vi "LSM9DS1 IMU Example.vi"() -> ()   [LabVIEW 2020]
doc: "Example for reading from the LSM9DS1 9-axis IMU using the LINX toolkit."
uses:
  <vilib>/MakerHub/LINX/Public/Utilities/Open Local.vi
  LINX I2C/LINX I2C.lvclass
  <vilib>/MakerHub/LINX/LMH-LINX.lvlib
  LSM9DS1/LSM9DS1 IMU.lvclass
panel:
  out "Magnetometer":cluster{"x":dbl, "y":dbl, "z":dbl}(graph)
  out "Accelerometer":cluster{"x":dbl, "y":dbl, "z":dbl}(graph)
  in  "stop":bool
  out "Gyro":cluster{"x":dbl, "y":dbl, "z":dbl}(graph)
  out "Error Out":errorcluster
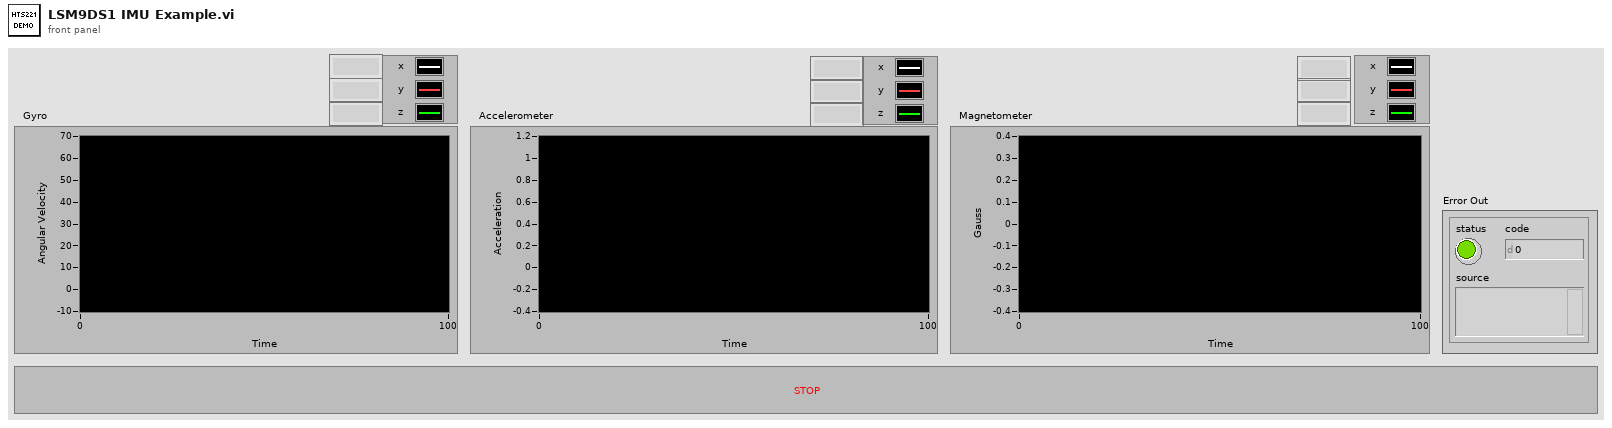
[diagram p1: front panel]
types:
  T1 = typedef "LMH-LINX.lvlib/LINX Ref.ctl" = cluster{"IO":T2, "Interface":T3, "LINX Device Config":T4}
  T2 = typedef "LMH-LINX.lvlib/Platform.ctl" = enum16{"Remote", "Local"}
  T3 = typedef "LMH-LINX.lvlib/Interface.ctl" = enum16{"Serial", "TCP"}
  T4 = typedef "LMH-LINX.lvlib/Device.lvlib/LINX Device Config.ctl" = cluster{"Interface":T3, "COM Port":refnum<visa-resource-name>, "TCP Configuration":T5, "Device Family":u8, "Device ID":u8, "Device Name":string, "TCP Ref":refnum<k5>, "Channels":T6}
  T5 = typedef "LMH-LINX.lvlib/Device.lvlib/TCP Config.ctl" = cluster{"IP Address":string, "Port":u16}
  T6 = typedef "LMH-LINX.lvlib/Channels.ctl" = cluster{"DI":u8[], "DO":u8[], "AI":u8[], "AO":u8[], "PWM":u8[], "QE":u8[], "UART":u8[], "I2C 2":u8[], "SPI":u8[], "CAN":u8[], "Servo":u8[], "AI Ref (V)":dbl, "AI Resolution (Bits)":u8, "AO Ref (V)":dbl, "AO Resolution (Bits)":u8}
  T7 = typedef "LSM9DS1 IMU.lvclass/3 Axis Values.ctl" = cluster{"x":dbl, "y":dbl, "z":dbl}
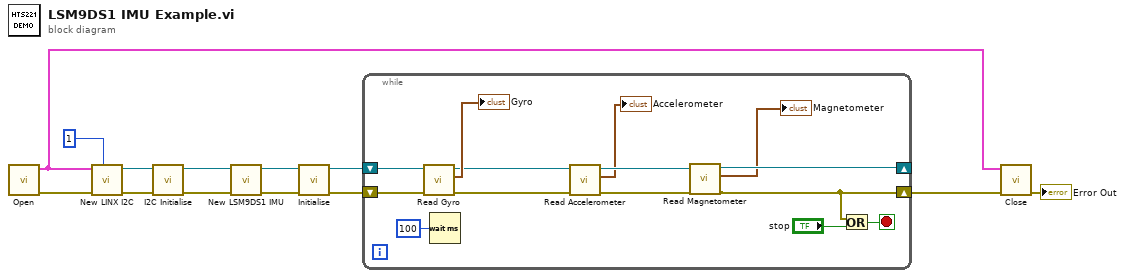
[diagram p0: block diagram]
diagram:
  n1 = call-poly <vilib>:"Open.vi"() -> ("Error Out"=w12:errorcluster, "LINX Resource"=w8:T1)  [unwired: 9 in, 1 out]
  n2 = call "New LINX I2C.vi"("LINX I2C Channel"=u8 1 ("I2C Channel"), "error in (no error)"=w12, "LINX Resource"=w8) -> ("error out"=w10:errorcluster, "LINX I2C out"=w9:refnum<class "LINX I2C.lvclass">)  [unwired: 7 in]
  n3 = call-dynamic "I2C Initialise.vi"("error in (no error)"=w10, "LINX I2C in"=w9) -> ("error out"=w5:errorcluster, "LINX I2C out"=w6:refnum<class "LINX I2C.lvclass">)  [unwired: 8 in]
  n4 = call "New LSM9DS1 IMU.vi"("error in (no error)"=w5, "I2C in"=w6) -> ("error out"=w3:errorcluster, "LSM9DS1 IMU out"=w4:refnum<class "LSM9DS1 IMU.lvclass">)  [unwired: 8 in]
  n5 = call "Initialise.vi"("error in (no error)"=w3, "LSM9DS1 IMU in"=w4) -> ("error out"=w1:errorcluster, "LSM9DS1 IMU out"=w2:refnum<class "LSM9DS1 IMU.lvclass">)  [unwired: 8 in]
  n6 = while {
    shift-right: [w16] -> w7
    shift-left: w1 -> [w23]
    shift-right: [w17] -> _
    shift-left: w2 -> [w24]
    stop <- w26 stop-if-true
    n7 = call "Read Gyro.vi"("error in (no error)"=w23, "LSM9DS1 IMU in"=w24) -> ("error out"=w20:errorcluster, "Gyro Values (dps)"=→"Gyro":T7, "LSM9DS1 IMU out"=w21:refnum<class "LSM9DS1 IMU.lvclass">)  [unwired: 7 in]
    n8 = Wait (ms)(milliseconds to wait=u32 100) -> ()  [unwired: 1 out]
    n9 = call "Read Accelerometer.vi"("error in (no error)"=w20, "LSM9DS1 IMU in"=w21) -> ("error out"=w19:errorcluster, "Accelerometer Values (g)"=→"Accelerometer":T7, "LSM9DS1 IMU out"=w18:refnum<class "LSM9DS1 IMU.lvclass">)  [unwired: 7 in]
    n10 = call "Read Magnetometer.vi"("error in (no error)"=w19, "LSM9DS1 IMU in"=w18) -> ("error out"=w16:errorcluster, "Magnetometer Values (gauss)"=→"Magnetometer":T7, "LSM9DS1 IMU out"=w17:refnum<class "LSM9DS1 IMU.lvclass">)  [unwired: 7 in]
    n11 = Or(x=w16, y="stop") -> (x .or. y?=w26:bool)
  }
  n12 = call <vilib>:"Close.vi"("Error In"=w7, "LINX Resource"=w8) -> ("Error Out"=→"Error Out":errorcluster)  [unwired: 9 in]
